vi "Power Module.vi"(0 "Calculate Analysis?":bool, 1 "Current Setpoint":dbl=3.0, 2 "Voltage Setpoint":dbl=6.0, 3 "Physical Channel":tag="PowerModule/power", 4 "error in":errorcluster) -> (25 "error out":errorcluster, 26 "Current Meas":dbl[](array[numeric]), 27 "Voltage Meas":dbl[](array[numeric]))   [LabVIEW 2021, in "Z Power Module Main Library.lvlib"]
uses:
  Power Measurement/Z Power Module Main Library.lvlib
  Power Measurement/Typedefs/Channel Settings.ctl
  Power Measurement/Typedefs/Timing Settings.ctl
  Power Measurement/Typedefs/Trigger Settings.ctl
  Power Measurement/Typedefs/Configure or Measure.ctl
  Power Measurement/Z Power Module Power Measurement.lvlib
panel:
  # "INPUT"
  # "OUTPUT"
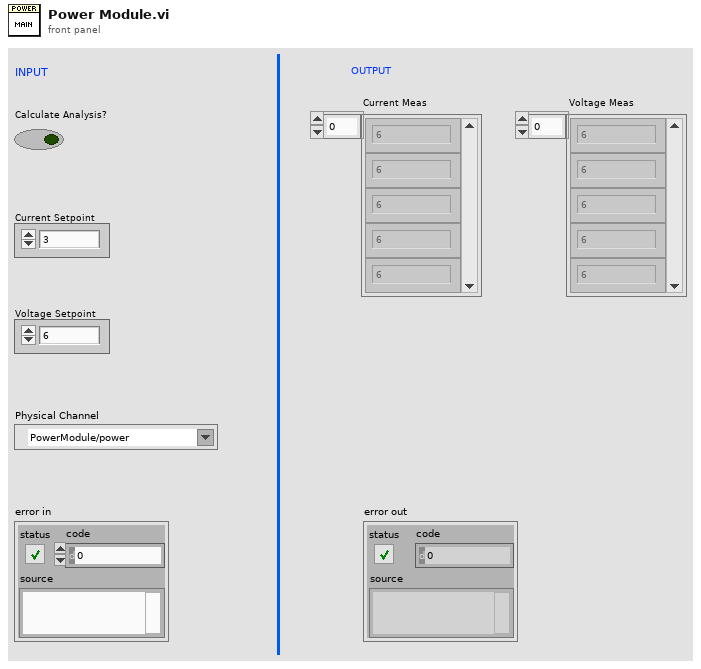
[diagram p1: front panel]
types:
  T1 = typedef "Z Power Module Power Measurement.lvlib/Configure or Measure.ctl" = enum16{"Configure Only", "Measure Only", "Configure and Measure"}
  T2 = typedef "Z Power Module Power Measurement.lvlib/Trigger Settings.ctl" = cluster{"Digital Start Trigger?":bool, "Digital Start Trigger Source":tag, "Digital Start Trigger Edge":i32}
  T3 = typedef "Z Power Module Power Measurement.lvlib/Timing Settings.ctl" = cluster{"Sample Clock Source":tag, "Sample Rate":dbl, "Number of Samples":i32}
  T4 = typedef "Z Power Module Power Measurement.lvlib/Channel Settings.ctl" = cluster{"Current Setpoint":dbl, "Voltage Setpoint":dbl}
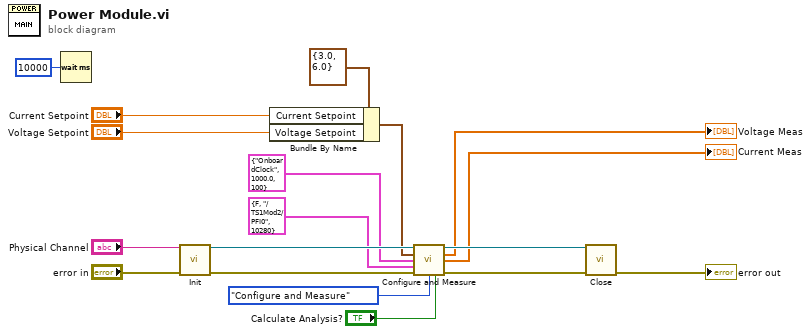
[diagram p0: block diagram]
diagram:
  n1 = Wait (ms)(milliseconds to wait=u32 10000) -> ()  [unwired: 1 out]
  n2 = call "Init.vi"("Physical Channel"="Physical Channel", "error in (no error)"="error in") -> ("task out"=w18:refnum<k21>, "error out"=w17:errorcluster)  [unwired: 12 in]
  n3 = Bundle By Name(cluster=T4 {"Current Setpoint"=3.0, "Voltage Setpoint"=6.0} ("Channel Settings"), "Current Setpoint"="Current Setpoint", "Voltage Setpoint"="Voltage Setpoint") -> (w8:T4)
  n4 = call "Configure and Measure.vi"("task/channels in"=w18, "Channel Settings"=w8, "Timing Settings"=T3 {"Sample Clock Source"="OnboardClock", "Sample Rate"=1000.0, "Number of Samples"=100}, "Trigger Settings"=T2 {"Digital Start Trigger?"=FALSE, "Digital Start Trigger Source"="/TS1Mod2/PFI0", "Digital Start Trigger Edge"=10280}, "error in (no error)"=w17, "Operation"=Configure_or_Measure."Configure and Measure", "Calculate Analysis?"="Calculate Analysis?") -> ("task out"=w15:refnum<k21>, "voltage"=→"Voltage Meas":dbl[], "Current"=→"Current Meas":dbl[], "error out"=w14:errorcluster)  [unwired: 4 in, 1 out]
  n5 = call "Close.vi"("task/channels in"=w15, "error in (no error)"=w14) -> ("error out"=→"error out":errorcluster)  [unwired: 13 in]
